vi "Populate.vi"(8 "error in (no error)":errorcluster, 10 "Data String":string, 11 "Project Builder in":refnum<class "Project Builder.lvclass">) -> (0 "error out":errorcluster, 3 "Project Builder out":refnum<class "Project Builder.lvclass">)   [LabVIEW 2020, in "ProjectBuilder.lvlib" / "Project Builder.lvclass"]
doc: "Populate Project Builder class from string.\n\nThe default implementation does nothing."
uses:
  Project Builder.lvclass
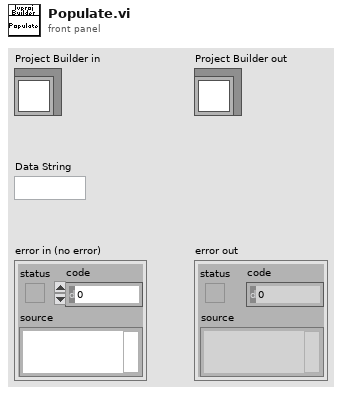
[diagram p1: front panel]
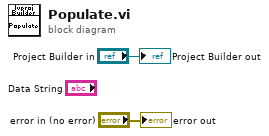
[diagram p0: block diagram]
diagram:
  "error out" <- "error in (no error)"
  "Project Builder out" <- "Project Builder in"
